vi "CAPTH-Init Data File.vi"(0 "Datafile path":path, 5 "Params":T1={"Stimulus"={"EAR"=enum."RIGHT", "HI FREQ"=18.0, "LO FREQ"=5.0, "FREQ STEP"=8, "Rep Rate (/s)"=20.0, "Alternate Polarity"=TRUE, "# CYCLES"=1, "Duration (ms)"=0.0, "Ramp (ms)"=0.0}, "Response"={"Averages (3dB steps)"=12, "Time Window (ms)"=8.5, "dt (us)"=10.0, "Grass gain"=1000.0, "CRITERION (mV)"=60.0, "CEILING (dB atten)"=6.0, "Use previous"=FALSE, "Save avgs"=FALSE, "Save raw"=FALSE, "Save history"=FALSE, "CEILING (dB SPL)"=6.0}} {"Response"."CRITERION (mV)" format="%.2f"; "Response"."Time Window (ms)" format="%.2f"}, 11 "error in (no error)":errorcluster) -> (15 "error out":errorcluster)   [LabVIEW 2020]
uses:
  Typedefs/CAPTH-Parameters.ctl
  Typedefs/CAPTH-Stimulus.ctl
  Typedefs/CAPTH-Response.ctl
  epl-vi-lib/Utility VIs/File IO VIs/Configuration File Wrapper VIs/Config-Read Key (string).vi
  <vilib>/regexp/Match Regular Expression.xnode
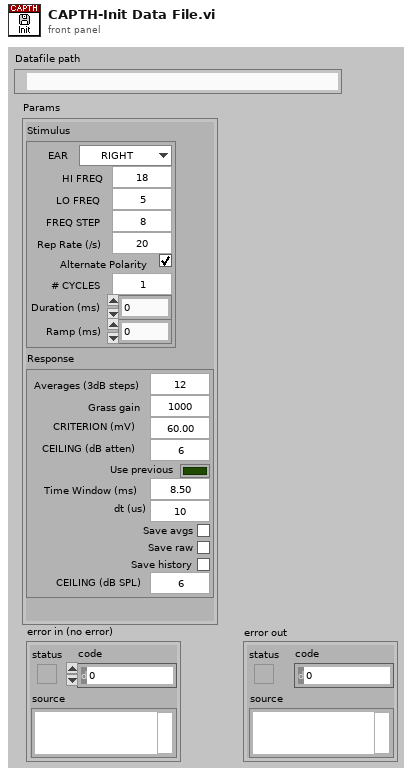
[diagram p1: front panel]
types:
  T1 = typedef "CAPTH-Parameters.ctl" = cluster{"Stimulus":T2, "Response":T3}
  T2 = typedef "CAPTH-Stimulus.ctl" = cluster{"EAR":enum16{"RIGHT", "LEFT\n", "ALTERNATE"}, "HI FREQ":dbl, "LO FREQ":dbl, "FREQ STEP":u8, "Rep Rate (/s)":dbl, "Alternate Polarity":bool, "# CYCLES":u8, "Duration (ms)":dbl, "Ramp (ms)":dbl}
  T3 = typedef "CAPTH-Response.ctl" = cluster{"Averages (3dB steps)":i32, "Time Window (ms)":dbl, "dt (us)":dbl, "Grass gain":dbl, "CRITERION (mV)":dbl, "CEILING (dB atten)":dbl, "Use previous":bool, "Save avgs":bool, "Save raw":bool, "Save history":bool, "CEILING (dB SPL)":dbl}
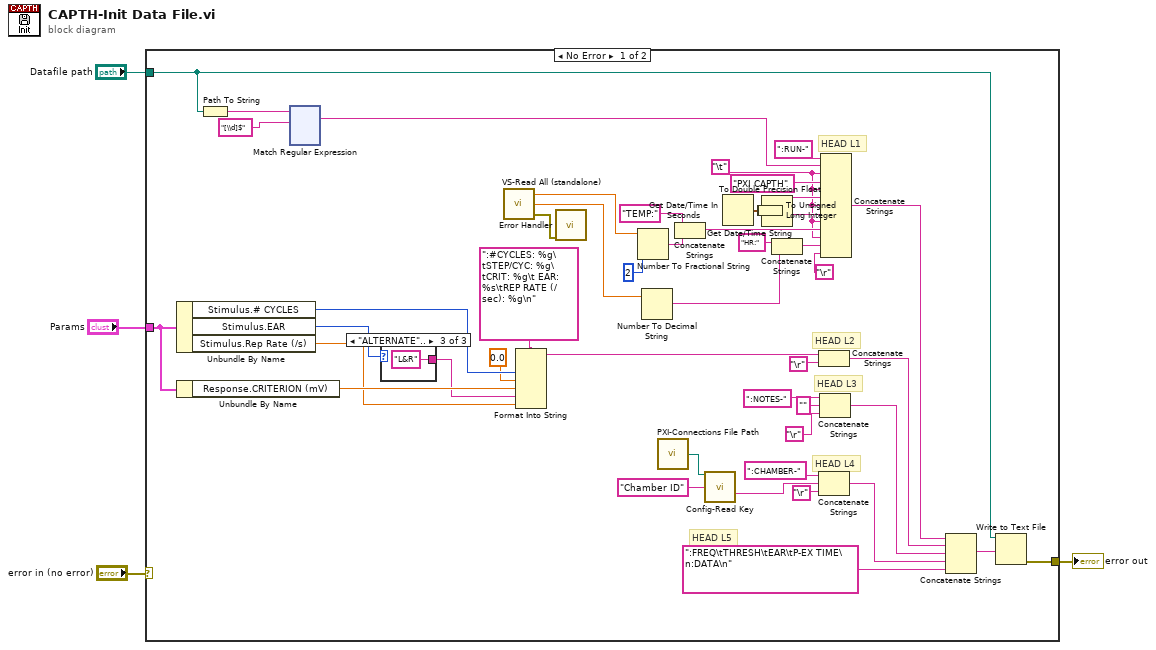
[diagram p0: block diagram]
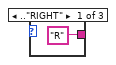
[diagram p2: hidden frame]
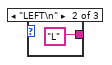
[diagram p3: hidden frame]
diagram:
  n1 = case shown="No Error" "error in (no error)" {
    selector: "error in (no error)" -> [_ w170]
    tunnel: [w26 w170] -> w4
    tunnel: "Datafile path" -> [w10 _]
    tunnel: "Params" -> [w11 _]
    frame No Error {
      w35 = "\t"
      # "HEAD L4"
      # "HEAD L5"
      # "HEAD L3"
      # "HEAD L2"
      # "HEAD L1"
      n2 = Unbundle By Name(w11) -> ("Stimulus.# CYCLES"=w23:u8, "Stimulus.EAR"=w20:enum16{"RIGHT", "LEFT\n", "ALTERNATE"}, "Stimulus.Rep Rate (/s)"=w18:dbl)
      n3 = Unbundle By Name(w11) -> ("Response.CRITERION (mV)"=w21:dbl)
      n4 = Path To String(path=w10) -> (string=w9:string)
      n5 = xnode "Match Regular Expression"("input string"=w9, "regular expression"="[\\d]$") -> ("whole match"=w7:string)  [unwired: 4 in, 4 out]
      n6 = case shown="\"ALTERNATE\".." w20 {
        tunnel: ["R" "L" "L&R"] -> w19
        frame .."RIGHT" {
        }
        frame "LEFT\n" {
        }
        frame "ALTERNATE".. {
        }
      }
      n7 = call "VS-Read All (standalone).vi"() -> ("error out"=w14:errorcluster, "Heart Rate (bpm)"=w15:dbl, "Temperature (C)"=w16:dbl)  [unwired: 3 in]
      n8 = Format Into String(format string=":#CYCLES: %g\tSTEP/CYC: %g\tCRIT: %g\t EAR: %s\tREP RATE (/sec): %g\n", w23, 0.0 ("input 2"), w21, w19, w18) -> (resulting string=w24:string)  [unwired: 2 in, 1 out]
      n9 = call "Error Handler.vi"("error in (no error)"=w14) -> ()  [unwired: 13 in, 2 out]
      n10 = Number To Fractional String(number=w16, precision (6)=2) -> (F-format string=w50:string)  [unwired: 2 in]
      n11 = Number To Decimal String(number=w15) -> (decimal integer string=w32:string)  [unwired: 1 in]
      n12 = call "PXI-Connections File Path.vi"() -> ("Path"=w5:path)  [unwired: 1 in]
      n13 = Concatenate Strings("TEMP:", w50) -> (w36:string)
      n14 = call-poly "Config-Read Key.vi"("configuration file path"=w5, "key"="Chamber ID" ("string")) -> ("value"=w6:string)  [unwired: 10 in, 3 out]
      n15 = Get Date/Time In Seconds() -> (seconds since 1Jan1904=w27:timestamp)
      n16 = To Double Precision Float(number=w27) -> (double precision float=w28:dbl)
      n17 = To Unsigned Long Integer(number=w28) -> (unsigned 32bit integer=w52:u32)
      n18 = Get Date/Time String(seconds (now)=w52) -> (date string=w38:string, time string=w37:string)  [unwired: 2 in]
      n19 = Concatenate Strings("HR:", w32) -> (w34:string)
      n20 = Concatenate Strings(w24, "\r") -> (w42:string)
      n21 = Concatenate Strings(":CHAMBER-", w6, "\r") -> (w29:string)
      n22 = Concatenate Strings(":NOTES-", "" ("string"), "\r") -> (w43:string)
      n23 = Concatenate Strings(":RUN-", w7, w35, "PXI CAPTH", w35, w38, w35, w37, w35, w36, w35, w34, "\r") -> (w41:string)
      n24 = Concatenate Strings(w41, w42, w43, w29, ":FREQ\tTHRESH\tEAR\tP-EX TIME\n:DATA\n") -> (w40:string)
      n25 = Write to Text File(file (use dialog)=w10, text=w40) -> (error out=w26:errorcluster)  [unwired: 2 in, 2 out]
    }
    frame Error {
    }
  }
  "error out" <- w4
